vi "Pause.vi"(8 "error in (no error)":errorcluster, 10 "Internal?":bool, 11 "Julabo FP-50 Settings":T1={"VISA resource name"="", "Simulated?"=FALSE, "Pump Power"=2} {"Pump Power" min=0 max=8 step=1}) -> (0 "error out":errorcluster, 3 "Julabo FP-50 Settings":T1={"VISA resource name"="", "Simulated?"=FALSE, "Pump Power"=2} {"Pump Power" min=0 max=8 step=1})   [LabVIEW 2018, in "Julabo Type FP-50 TCU.lvlib"]
uses:
  Julabo Type FP-50 TCU.lvlib
  Julabo FP-50 Settings.ctl
  Third Party Drivers/Julabo Type 1/JULABO DeviceDriver/JULABO DeviceDriver.lvlib
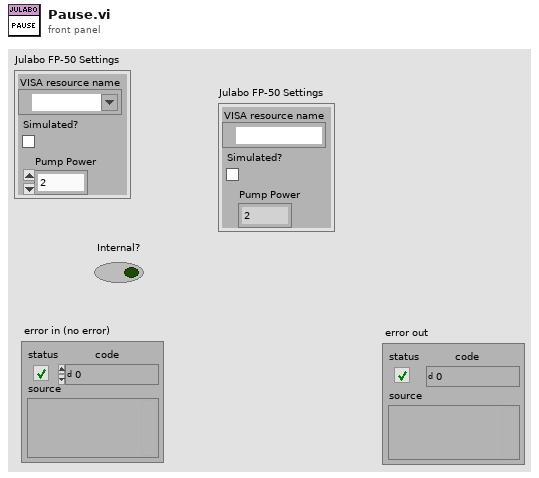
[diagram p1: front panel]
types:
  T1 = typedef "Julabo Type FP-50 TCU.lvlib/Julabo FP-50 Settings.ctl" = cluster{"VISA resource name":refnum<visa-resource-name>, "Simulated?":bool, "Pump Power":i32}
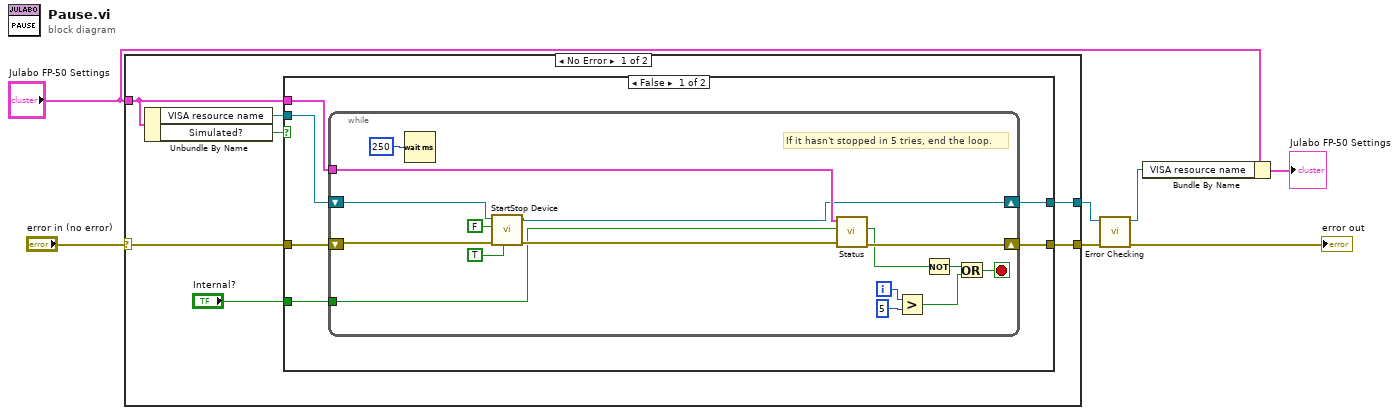
[diagram p0: block diagram]
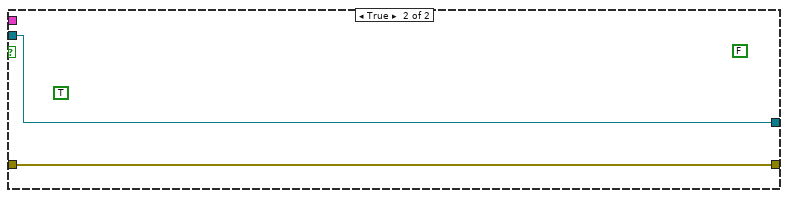
[diagram p2: hidden frame]
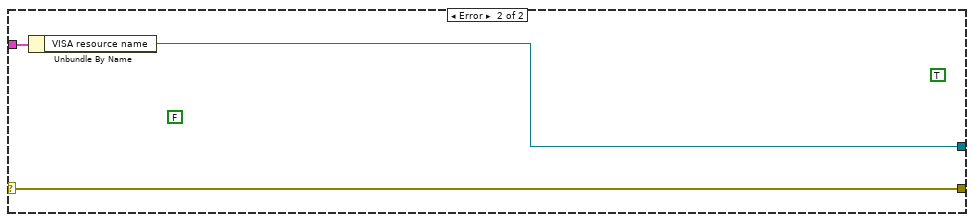
[diagram p3: hidden frame]
diagram:
  n1 = case shown="No Error" "error in (no error)" {
    selector: "error in (no error)" -> [w14 w41]
    tunnel: "Julabo FP-50 Settings" -> [w9 w40]
    tunnel: [w13 w41] -> w5
    tunnel: [w11 w39] -> w6
    frame No Error {
      n2 = Unbundle By Name(w9) -> ("VISA resource name"=w12:refnum<visa-resource-name>, "Simulated?"=w10:bool)
      n3 = case shown="False" w10 {
        tunnel: w14 -> [w18 w38]
        tunnel: [w16 w38] -> w13
        tunnel: [w20 w37] -> w11
        tunnel: w12 -> [w19 w37]
        tunnel: w9 -> [w17 _]
        tunnel: "Internal?" -> [w15 _]
        frame False {
          n4 = while {
            tunnel: w17 -> [w36]
            shift-right: [w23] -> w20
            shift-left: w19 -> [w26]
            shift-right: [w35] -> w16
            shift-left: w18 -> [w25]
            tunnel: w15 -> [w22]
            i -> [w33]
            stop <- w34 stop-if-true
            # "If it hasn't stopped in 5 tries, end the loop."
            n5 = Wait (ms)(milliseconds to wait=u32 250) -> ()  [unwired: 1 out]
            n6 = call "StartStop Device.vi"("parseError? T:Yes"=TRUE, "error in (no error)"=w25, "Start/Stop (f:Stop)"=FALSE, "VISA resource name"=w26) -> ("error out"=w24:errorcluster, "VISA resource name out"=w23:refnum<visa-resource-name>)  [unwired: 6 in]
            n7 = call "Status.vi"("error in (no error)"=w24, "Internal?"=w22, "Julabo FP-50 Settings"=w36) -> ("error out"=w35:errorcluster, "Running"=w28:bool)  [unwired: 3 in, 4 out]
            n8 = Greater?(x=w33, y=5) -> (0:w31:bool)
            n9 = Not(x=w28) -> (.not. x?=w29:bool)
            n10 = Or(x=w29, y=w31) -> (x .or. y?=w34:bool)
          }
        }
        frame True {
          (unwired) TRUE
          (unwired) FALSE
        }
      }
    }
    frame Error {
      (unwired) FALSE
      (unwired) TRUE
      n11 = Unbundle By Name(w40) -> ("VISA resource name"=w39:refnum<visa-resource-name>)
    }
  }
  n12 = call "Error Checking.vi"("error in (no error)"=w5, "VISA resource name"=w6) -> ("error out"=→"error out":errorcluster, "VISA resource name"=w3:refnum<visa-resource-name>)  [unwired: 7 in, 1 out]
  n13 = Bundle By Name(cluster="Julabo FP-50 Settings", "VISA resource name"=w3) -> (→"Julabo FP-50 Settings":T1)
